vi "Create All Message Queues (OPC).vi"(8 "error in (no error)":errorcluster, 11 "Process Name":string) -> (0 "error out":errorcluster, 3 "Message Queues":T1)   [LabVIEW 2018, in "OPC UA.lvlib"]
uses:
  OPC UA.lvlib
  Message Queues.ctl
  support/Message Queue/Message Cluster.ctl
  OPC Display Cluster.ctl
  support/Message Queue/Enqueue Message (Single).vi
  support/Message Queue/Message Queue.lvlib
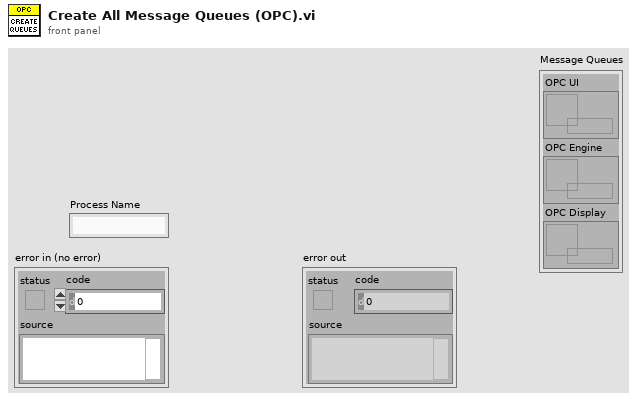
[diagram p1: front panel]
types:
  T1 = typedef "OPC UA.lvlib/Message Queues.ctl" = cluster{"OPC UI":refnum<queue>, "OPC Engine":refnum<queue>, "OPC Display":refnum<queue>}
  T2 = typedef "OPC UA.lvlib/OPC Display Cluster.ctl" = cluster{"URL":string, "Cycle":i32, "Updating":bool}
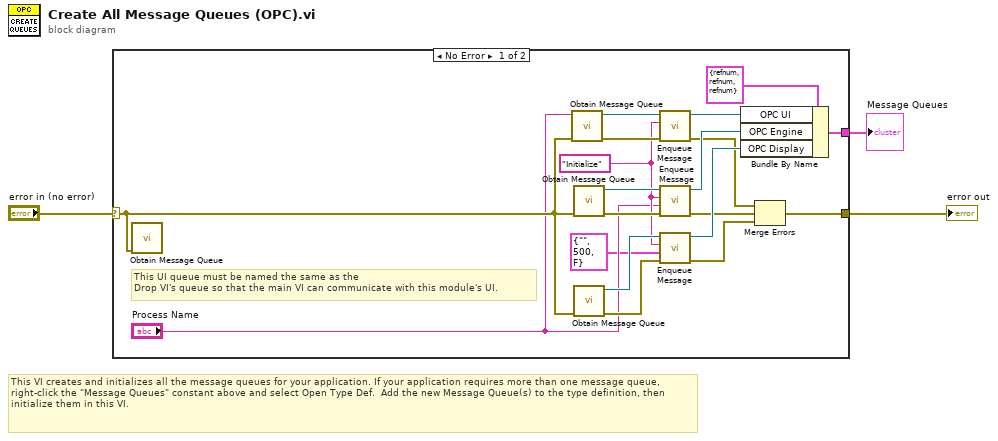
[diagram p0: block diagram]
diagram:
  # "This VI creates and initializes all the message queues for your application. If your application requires more than one message queue, right-click the \"Message Queues\" constant above and select Open Type Def.  Add the new Message Queue(s) to the type definition, then initialize them in this VI."
  n1 = case shown="No Error" "error in (no error)" {
    selector: "error in (no error)" -> [w8 w23]
    tunnel: [w21 w23] -> w3
    tunnel: [w22 _] -> w1
    frame No Error {
      w7 = "Initialize" ("Message")
      # "This UI queue must be named the same as the \nDrop VI's queue so that the main VI can communicate with this module's UI."
      n2 = call "Obtain Message Queue.vi"("error in (no error)"=w8) -> ()  [unwired: 9 in, 2 out]
      n3 = call "Obtain Message Queue.vi"("error in (no error)"=w8, "name (unnamed)"="Process Name") -> ("error out"=w17:errorcluster, "Message Queue"=w20:refnum<queue>)  [unwired: 8 in]
      n4 = call "Obtain Message Queue.vi"("error in (no error)"=w8) -> ("error out"=w16:errorcluster, "Message Queue"=w19:refnum<queue>)  [unwired: 9 in]
      n5 = call "Obtain Message Queue.vi"("error in (no error)"=w8) -> ("error out"=w15:errorcluster, "Message Queue"=w18:refnum<queue>)  [unwired: 9 in]
      n6 = call-poly "Enqueue Message.vi"("error in (no error)"=w17, "Message"=w7, "Message Queue"=w20) -> ("error out"=w11:errorcluster, "dup Message Queue"=w14:refnum<queue>)  [unwired: 7 in]
      n7 = call-poly "Enqueue Message.vi"("error in (no error)"=w16, "Message Data"="Process Name", "Message"=w7, "Message Queue"=w19) -> ("error out"=w10:errorcluster, "dup Message Queue"=w13:refnum<queue>)  [unwired: 6 in]
      n8 = call-poly "Enqueue Message.vi"("error in (no error)"=w15, "Message Data"=T2 {"URL"="", "Cycle"=500, "Updating"=FALSE} ("OPC Display Cluster"), "Message"=w7, "Message Queue"=w18) -> ("error out"=w9:errorcluster, "dup Message Queue"=w12:refnum<queue>)  [unwired: 6 in]
      n9 = Bundle By Name(cluster=T1 {"OPC UI"=refnum, "OPC Engine"=refnum, "OPC Display"=refnum} ("Message Queues"), "OPC UI"=w14, "OPC Engine"=w13, "OPC Display"=w12) -> (w22:T1)
      n10 = Merge Errors(w11, w10, w9) -> (w21:errorcluster)
    }
    frame Error {
    }
  }
  "error out" <- w3
  "Message Queues" <- w1
